vi "Get Plot to Fit Wrapper.vi"(6 "Clip Plot? (True)":bool=TRUE, 8 "error in (no error)":errorcluster, 11 "Fit Plot Information":T2) -> (0 "error out":errorcluster, 1 "Plot Color":u32, 2 "Plot Name":string, 3 "Clipped Plot":T1, 4 "Graph Name":string, 5 "Full Plot":T1, 7 "Fit Model":T4)   [LabVIEW 2021, in "Fits.lvlib"]
uses:
  Fits.lvlib
  Graphs/Graphs.lvlib
  Graphs/Get Plot at Mouse Click (XY Graph)/Get Plot at Mouse Click [AAC].vi
  Fit Models.ctl
  <vilib>/Utility/miscctls.llb/LVPointDoubleTypeDef.ctl
  Fit Plot Request Information.ctl
  Graphs/XY Graph/XY Graph Plot Data.ctl
  Graphs/XY Graph/XY Graph Add-Ons.lvlib
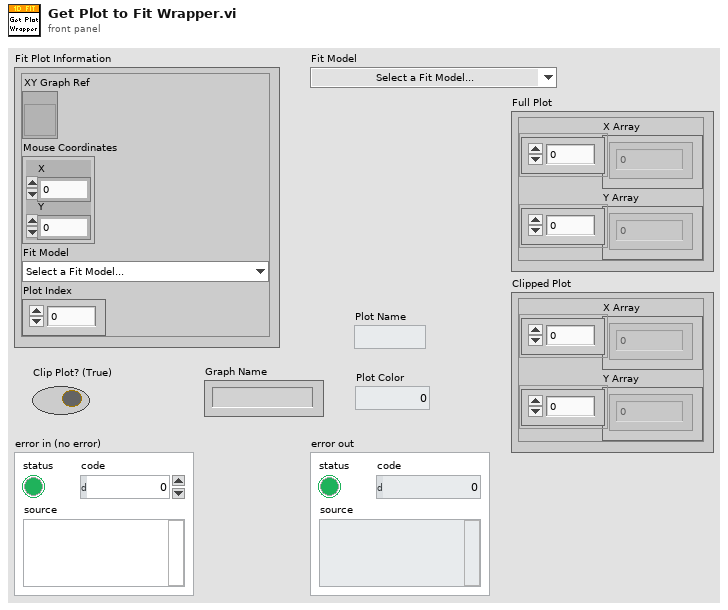
[diagram p1: front panel]
types:
  T1 = typedef "XY Graph Add-Ons.lvlib/XY Graph Plot Data.ctl" = cluster{"X Array":dbl[], "Y Array":dbl[]}
  T2 = typedef "Fits.lvlib/Fit Plot Request Information.ctl" = cluster{"XY Graph Ref":refnum<vi>, "Mouse Coordinates":T3, "Fit Model":T4, "Plot Index":i32}
  T3 = typedef "LVPointDoubleTypeDef.ctl" = cluster{"X":dbl, "Y":dbl}
  T4 = typedef "Fits.lvlib/Fit Models.ctl" = enum16{"Select a Fit Model...", "           Single Peak", "Gaussian", "Asymmetric Gaussian", "Lorentzian", "Asymmetric Lorentzian", "Gaussian/Lorentzian", "Lorentzian/Gaussian", "           Double Peak", "Two Gaussians", "Two Asymmetric Gaussians", "Two H-Connected Gaussians", "Two T-Connected Gaussians", "Two H-Connected Asymmetric Gaussians", "Two T-Connected Asymmetric Gaussians", "           Triple Peak", "Three Gaussians", "Three Asymmetric Gaussians", "              Decays", "1-Exponential", "IRF*PSED", "2-Exponentials", "            Power Law", "Power Law", "Power Law with Offset", "               ACF", "2D Gaussian ACF", "2D Gaussian + Blinking ACF", "2D Gaussian + Flow ACF", "3D Gaussian ACF", "3D Gaussian + Blinking ACF", "             Multiplot", "2D Gaussian ACF & 2D Gaussian + Flow ACF"}
  T5 = typedef "XY Graph Add-Ons.lvlib/XY Graph Refnum.ctl" = refnum<vi>
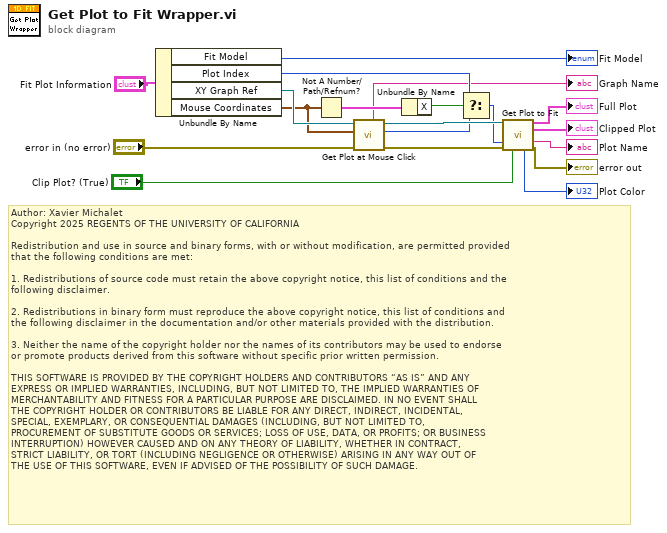
[diagram p0: block diagram]
diagram:
  # "Author: Xavier Michalet\nCopyright 2025 REGENTS OF THE UNIVERSITY OF CALIFORNIA\n\nRedistribution and use in source and binary forms, with or without modification, are permitted provided\nthat the following conditions are met:\n\n1. Redistributions of source code must retain the above copyright notice, this list of conditions and the\nfollowing disclaimer.\n\n2. Redistributions in binary form must reproduce the above copyright notice, this list of conditions and\nthe following disclaimer in the documentation and/or other materials provided with the distribution.\n\n3. Neither the name of the copyright holder nor the names of its contributors may be used to endorse \nor promote products derived from this software without specific prior written permission.\n\nTHIS SOFTWARE IS PROVIDED BY THE COPYRIGHT HOLDERS AND CONTRIBUTORS “AS IS” AND ANY \nEXPRESS OR IMPLIED WARRANTIES, INCLUDING, BUT NOT LIMITED TO, THE IMPLIED WARRANTIES OF\nMERCHANTABILITY AND FITNESS FOR A PARTICULAR PURPOSE ARE DISCLAIMED. IN NO EVENT SHALL\nTHE COPYRIGHT HOLDER OR CONTRIBUTORS BE LIABLE FOR ANY DIRECT, INDIRECT, INCIDENTAL, \nSPECIAL, EXEMPLARY, OR CONSEQUENTIAL DAMAGES (INCLUDING, BUT NOT LIMITED TO, \nPROCUREMENT OF SUBSTITUTE GOODS OR SERVICES; LOSS OF USE, DATA, OR PROFITS; OR BUSINESS\nINTERRUPTION) HOWEVER CAUSED AND ON ANY THEORY OF LIABILITY, WHETHER IN CONTRACT, \nSTRICT LIABILITY, OR TORT (INCLUDING NEGLIGENCE OR OTHERWISE) ARISING IN ANY WAY OUT OF\nTHE USE OF THIS SOFTWARE, EVEN IF ADVISED OF THE POSSIBILITY OF SUCH DAMAGE."
  n1 = Unbundle By Name("Fit Plot Information") -> ("Fit Model"=→"Fit Model":T4, "Plot Index"=w6:i32, "XY Graph Ref"=w14:refnum<vi>, "Mouse Coordinates"=w5:T3)
  n2 = Not A Number/Path/Refnum?(number/path/refnum=w5) -> (NaN/Path/Refnum?=w10:cluster{"X":bool, "Y":bool})
  n3 = call-poly "Get Plot at Mouse Click.vi"("error in (no error)"="error in (no error)", "Mouse Click Coordinates"=w5, "XY Graph in"=w14) -> ("error out"=w15:errorcluster, "Plot at Coordinates"=w8:i32, "XY Graph out"=w19:T5, "Graph Name"=→"Graph Name":string)  [unwired: 2 in, 3 out]
  n4 = Unbundle By Name(w10) -> ("X"=w9:bool)
  n5 = Select(t=w6, s=w9, f=w8) -> (s? t:f=w16:i32)
  n6 = call "Get Plot to Fit.vi"("XYGraph in"=w19, "Plot Index"=w16, "error in (no error)"=w15, "Clip Plot? (True)"="Clip Plot? (True)") -> ("Full Plot"=→"Full Plot":T1, "Clipped Plot"=→"Clipped Plot":T1, "Plot Name"=→"Plot Name":string, "Plot Color"=→"Plot Color":u32, "error out"=→"error out":errorcluster)  [unwired: 5 in, 2 out]
